vi "Mischer_LevelmeterMonitor.vi"() -> ()   [LabVIEW 2018]
uses:
  Utility/Monitor Communication/Mischer/Mischer_Levelmeter-Cluster.ctl
  Instrument_Setup.vi
  Global/Global Variables/Data_Display_global.vi
panel:
  in  "Stopp":bool
  in  "Mischer Levelmeter":T1={"Plot"=[], "N-Shield (%)"=0.0, "He (%)"=0.0, "Coldtrap (%)"=0.0, "He - POT (%)"=0.0, "N-Shield Refill"=FALSE, "Last fill Shield"="", "Auto Refill Shield"=TRUE, "Trap Refill"=FALSE, "Last fill Coldtrap"="", "Auto Refill Trap"=TRUE, "Shield Refill"=FALSE, "Coldtrap Refill"=FALSE, "Auto Trap activatet"=FALSE, "Auto Shield Activatet"=FALSE}
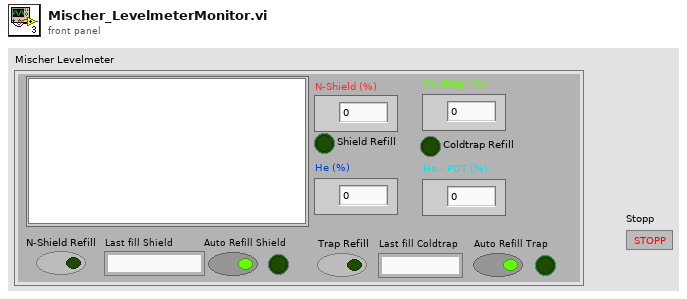
[diagram p1: front panel]
types:
  T1 = typedef "Mischer_Levelmeter-Cluster.ctl" = cluster{"Plot":dbl[][], "N-Shield (%)":dbl, "He (%)":dbl, "Coldtrap (%)":dbl, "He - POT (%)":dbl, "N-Shield Refill":bool, "Last fill Shield":string, "Auto Refill Shield":bool, "Trap Refill":bool, "Last fill Coldtrap":string, "Auto Refill Trap":bool, "Shield Refill":bool, "Coldtrap Refill":bool, "Auto Trap activatet":bool, "Auto Shield Activatet":bool}
  T2 = cluster{"Arduino Levelmeter":refnum<visa-resource-name>, "TIC Comport":refnum<visa-resource-name>}
  T3 = typedef "Mischer_Levelmeter_Control.ctl" = cluster{"N-Shield Refill":bool, "Automatic Refill Shield":bool, "Trap Refill":bool, "Automatic Refill Trap":bool}
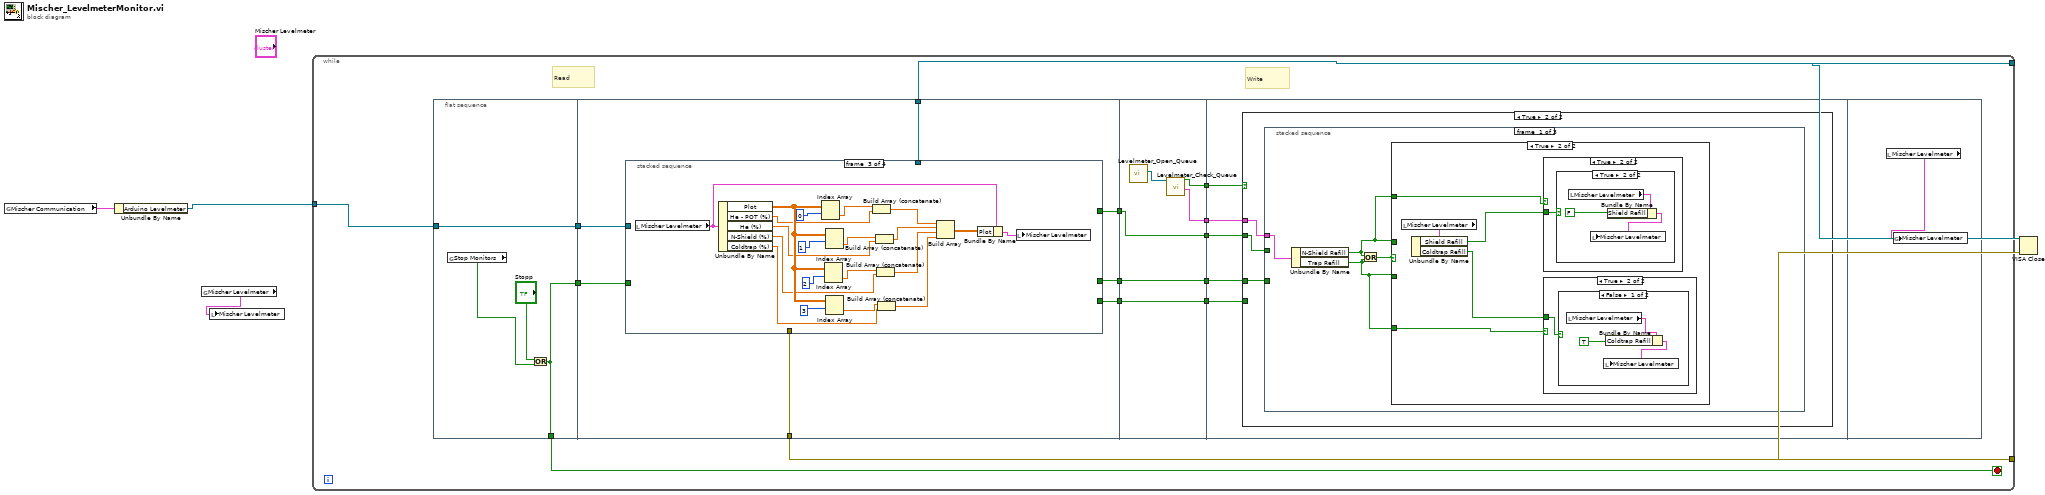
[diagram p0: block diagram]
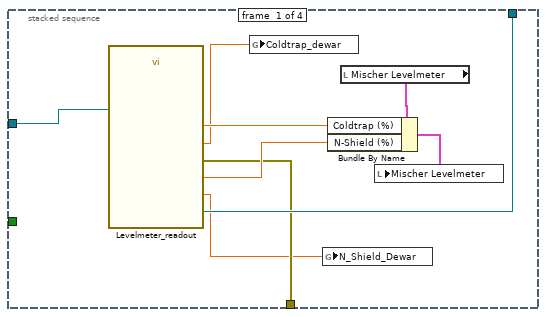
[diagram p2: hidden frame]
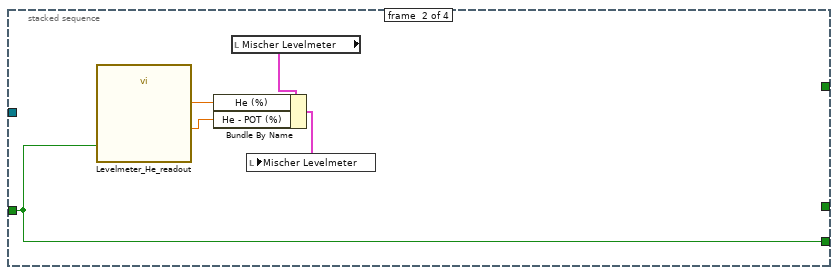
[diagram p3: hidden frame]
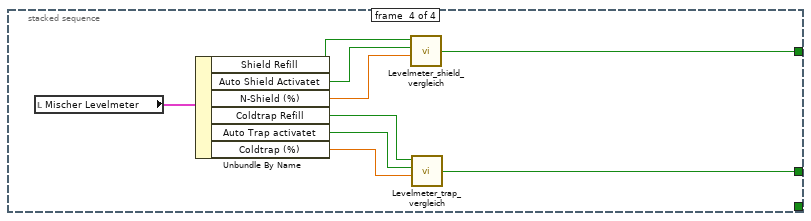
[diagram p4: hidden frame]
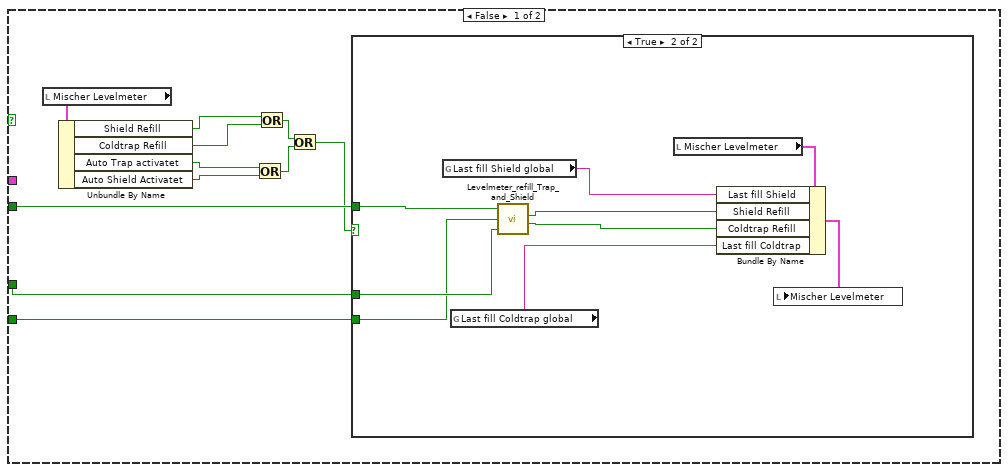
[diagram p5: hidden frame]
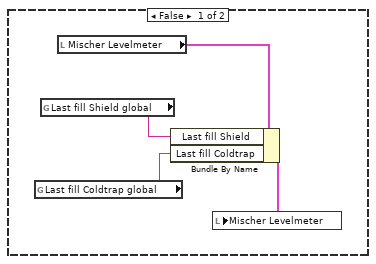
[diagram p6: hidden frame]
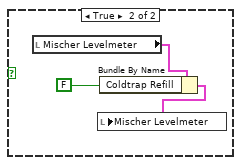
[diagram p9: hidden frame]
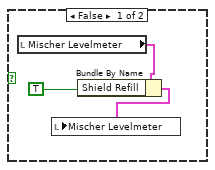
[diagram p11: hidden frame]
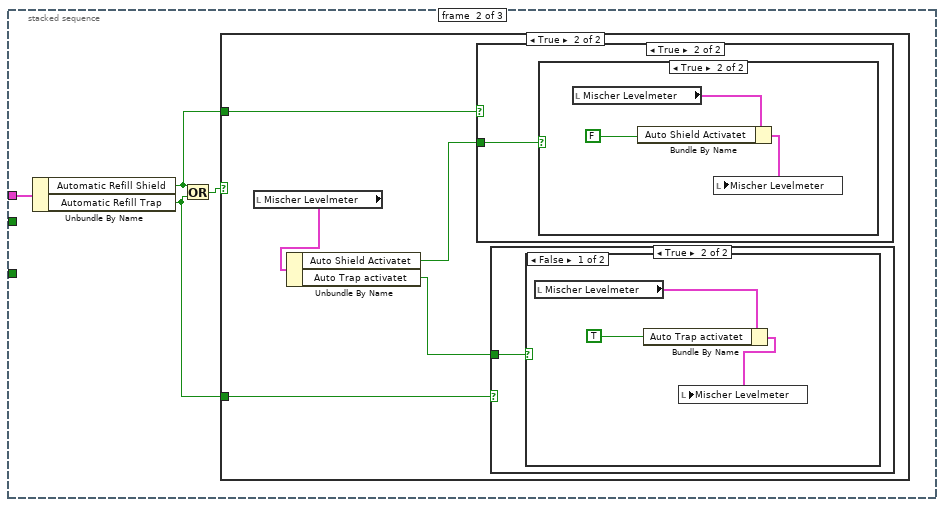
[diagram p12: hidden frame]
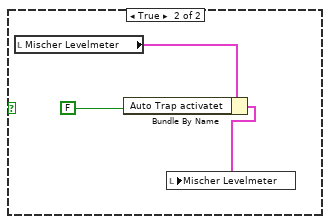
[diagram p15: hidden frame]
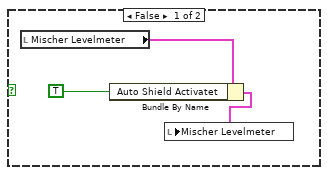
[diagram p17: hidden frame]
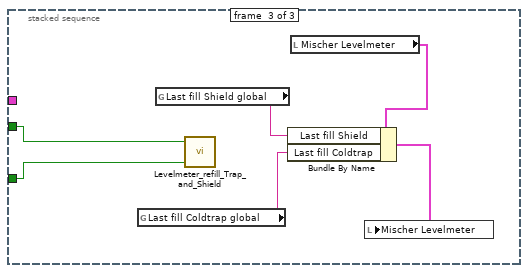
[diagram p18: hidden frame]
diagram:
  n1 = global read "Instrument_Setup.vi" "Mischer Communication"() -> (w5:T2)
  n2 = Unbundle By Name(w5) -> ("Arduino Levelmeter"=w1:refnum<visa-resource-name>)
  n3 = global read "Data_Display_global.vi" "Mischer Levelmeter"() -> (w4:T1)
  n4 = local write "Mischer Levelmeter"(w4) -> ()
  n5 = while {
    tunnel: w1 -> [w19]
    tunnel: [w12] -> w3
    tunnel: [w11] -> w2
    stop <- w9 stop-if-true
    # "Write"
    # "Read"
    n6 = flat-sequence {
      tunnel: w19 -> [w23]
      tunnel: [w23] -> w10
      tunnel: [w20] -> w9
      tunnel: [w20] -> w8
      tunnel: [w29] -> w16
      tunnel: [w28] -> w15
      tunnel: [w27] -> w12
      tunnel: [w26] -> w11
      tunnel: w10 -> [w30]
      tunnel: w8 -> [w25]
      tunnel: [w24] -> w6
      tunnel: [w78] -> w18
      tunnel: [w77] -> w17
      tunnel: w16 -> [w76]
      tunnel: w15 -> [w75]
      tunnel: [w76] -> w14
      tunnel: [w75] -> w13
      tunnel: [w74] -> w7
      tunnel: w6 -> [w74]
      tunnel: w18 -> [w83]
      tunnel: w17 -> [w84]
      tunnel: w14 -> [w82]
      tunnel: w13 -> [w81]
      tunnel: w7 -> [w80]
      frame #0 {
        n7 = global read "Data_Display_global.vi" "Stop Monitors"() -> (w22:bool)
        n8 = Or(x="Stopp", y=w22) -> (x .or. y?=w20:bool)
      }
      frame #1 {
        n9 = stacked-sequence {
          tunnel: w30 -> [w39 _ _ _]
          tunnel: [_ _ _ w65] -> w29
          tunnel: [_ _ _ w66] -> w28
          tunnel: [w34 _ _ _] -> w27
          tunnel: [w33 _ _ _] -> w26
          tunnel: w25 -> [_ w40 _ _]
          tunnel: [_ w40 _ _] -> w24
          frame #0 {
            n10 = call "Levelmeter_readout.vi"("VISA-Ressourcenname"=w39) -> ("LN Shield Dewar [%]"=w31:dbl, "Coldtrap Dewar [%]"=w32:dbl, "Cold trap [%]"=w36:dbl, "LN Shield [%]"=w35:dbl, "VISA-Ressourcenname 2"=w34:refnum<visa-resource-name>, "error out"=w33:errorcluster)  [unwired: 4 in]
            n11 = global write "Data_Display_global.vi" "Coldtrap_dewar"(w32) -> ()
            n12 = global write "Data_Display_global.vi" "N_Shield_Dewar"(w31) -> ()
            n13 = local read "Mischer Levelmeter"() -> (w38:T1)
            n14 = Bundle By Name(cluster=w38, "Coldtrap (%)"=w36, "N-Shield (%)"=w35) -> (w37:T1)
            n15 = local write "Mischer Levelmeter"(w37) -> ()
          }
          frame #1 {
            n16 = call "Levelmeter_He_readout.vi"("stop DAQ"=w40) -> ("He-Pot in (%)"=w41:dbl, "He Bath (%)"=w44:dbl)  [unwired: 9 in]
            n17 = local read "Mischer Levelmeter"() -> (w43:T1)
            n18 = Bundle By Name(cluster=w43, "He (%)"=w44, "He - POT (%)"=w41) -> (w42:T1)
            n19 = local write "Mischer Levelmeter"(w42) -> ()
          }
          frame #2 {
            n20 = local read "Mischer Levelmeter"() -> (w47:T1)
            n21 = Unbundle By Name(w47) -> ("Plot"=w64:dbl[][], "He - POT (%)"=w58:dbl, "He (%)"=w56:dbl, "N-Shield (%)"=w54:dbl, "Coldtrap (%)"=w52:dbl)
            n22 = Index Array(array=w64, index (row)=0) -> (element=w59:dbl[])  [unwired: 1 in]
            n23 = Index Array(array=w64, index (row)=2) -> (element=w55:dbl[])  [unwired: 1 in]
            n24 = Index Array(array=w64, index (row)=1) -> (element=w57:dbl[])  [unwired: 1 in]
            n25 = Index Array(array=w64, index (row)=3) -> (element=w53:dbl[])  [unwired: 1 in]
            n26 = Build Array (concatenate)(w59, w58) -> (w51:dbl[])
            n27 = Build Array (concatenate)(w57, w56) -> (w50:dbl[])
            n28 = Build Array (concatenate)(w55, w54) -> (w49:dbl[])
            n29 = Build Array (concatenate)(w53, w52) -> (w48:dbl[])
            n30 = Build Array(w51, w50, w49, w48) -> (w46:dbl[][])
            n31 = Bundle By Name(cluster=w47, "Plot"=w46) -> (w45:T1)
            n32 = local write "Mischer Levelmeter"(w45) -> ()
          }
          frame #3 {
            n33 = local read "Mischer Levelmeter"() -> (w67:T1)
            n34 = Unbundle By Name(w67) -> ("Shield Refill"=w73:bool, "Auto Shield Activatet"=w72:bool, "N-Shield (%)"=w71:dbl, "Coldtrap Refill"=w70:bool, "Auto Trap activatet"=w69:bool, "Coldtrap (%)"=w68:dbl)
            n35 = call "Levelmeter_shield_vergleich.vi"("Shield Level (%)"=w71, "Automatic Shield refill activatet"=w72, "LN Shield Refill activatet"=w73) -> ("Data out"=w65:bool)  [unwired: 3 in]
            n36 = call "Levelmeter_trap_vergleich.vi"("Coldtrap Level (%)"=w68, "Automatic Trap refill activatet"=w69, "LN trap Refill activatet"=w70) -> ("Data out"=w66:bool)  [unwired: 3 in]
          }
        }
      }
      frame #2 {
        n37 = call "Levelmeter_Open_Queue.vi"() -> ("queue out"=w79:refnum<queue>)  [unwired: 10 in, 1 out]
        n38 = call "Levelmeter_Check_Queue.vi"("queue"=w79) -> ("Mischer Levelmeter  Control"=w78:T3, "New Entries?"=w77:bool)  [unwired: 7 in, 1 out]
      }
      frame #3 {
        n39 = case shown="True" w84 {
          tunnel: w83 -> [_ w111]
          tunnel: w82 -> [w95 w110]
          tunnel: w81 -> [w94 w109]
          tunnel: w80 -> [w85 _]
          frame False {
            n40 = local read "Mischer Levelmeter"() -> (w93:T1)
            n41 = Unbundle By Name(w93) -> ("Shield Refill"=w92:bool, "Coldtrap Refill"=w91:bool, "Auto Trap activatet"=w90:bool, "Auto Shield Activatet"=w89:bool)
            n42 = Or(x=w90, y=w89) -> (x .or. y?=w87:bool)
            n43 = Or(x=w92, y=w91) -> (x .or. y?=w88:bool)
            n44 = Or(x=w88, y=w87) -> (x .or. y?=w86:bool)
            n45 = case shown="True" w86 {
              tunnel: w95 -> [_ w108]
              tunnel: w94 -> [_ w107]
              tunnel: w85 -> [_ w100]
              frame False {
                n46 = global read "Data_Display_global.vi" "Last fill Coldtrap global"() -> (w96:string)
                n47 = global read "Data_Display_global.vi" "Last fill Shield global"() -> (w97:string)
                n48 = local read "Mischer Levelmeter"() -> (w99:T1)
                n49 = Bundle By Name(cluster=w99, "Last fill Shield"=w97, "Last fill Coldtrap"=w96) -> (w98:T1)
                n50 = local write "Mischer Levelmeter"(w98) -> ()
              }
              frame True {
                n51 = global read "Data_Display_global.vi" "Last fill Shield global"() -> (w102:string)
                n52 = global read "Data_Display_global.vi" "Last fill Coldtrap global"() -> (w101:string)
                n53 = call "Levelmeter_refill_Trap_and_Shield.vi"("Shield Refill"=w108, "Stop DAQ"=w100, "Trap Refill"=w107) -> ("Shield control"=w105:bool, "Trap control"=w104:bool)  [unwired: 2 in]
                n54 = local read "Mischer Levelmeter"() -> (w106:T1)
                n55 = Bundle By Name(cluster=w106, "Last fill Shield"=w102, "Shield Refill"=w105, "Coldtrap Refill"=w104, "Last fill Coldtrap"=w101) -> (w103:T1)
                n56 = local write "Mischer Levelmeter"(w103) -> ()
              }
            }
          }
          frame True {
            n57 = stacked-sequence {
              tunnel: w111 -> [w114 w138 _]
              tunnel: w110 -> [_ _ w163]
              tunnel: w109 -> [_ _ w162]
              frame #0 {
                n58 = Unbundle By Name(w114) -> ("N-Shield Refill"=w113:bool, "Trap Refill"=w112:bool)
                n59 = Or(x=w113, y=w112) -> (x .or. y?=w115:bool)
                n60 = case shown="True" w115 {
                  tunnel: w113 -> [_ _]
                  tunnel: w112 -> [_ _]
                  tunnel: w113 -> [_ w119]
                  tunnel: w112 -> [_ w118]
                  frame False {
                  }
                  frame True {
                    n61 = local read "Mischer Levelmeter"() -> (w120:T1)
                    n62 = Unbundle By Name(w120) -> ("Shield Refill"=w117:bool, "Coldtrap Refill"=w116:bool)
                    n63 = case shown="True" w119 {
                      tunnel: w117 -> [_ w128]
                      frame False {
                      }
                      frame True {
                        n64 = case shown="True" w128 {
                          frame False {
                            n65 = local read "Mischer Levelmeter"() -> (w131:T1)
                            n66 = Bundle By Name(cluster=w131, "Shield Refill"=TRUE) -> (w130:T1)
                            n67 = local write "Mischer Levelmeter"(w130) -> ()
                          }
                          frame True {
                            n68 = local read "Mischer Levelmeter"() -> (w134:T1)
                            n69 = Bundle By Name(cluster=w134, "Shield Refill"=FALSE) -> (w133:T1)
                            n70 = local write "Mischer Levelmeter"(w133) -> ()
                          }
                        }
                      }
                    }
                    n71 = case shown="True" w118 {
                      tunnel: w116 -> [_ w121]
                      frame False {
                      }
                      frame True {
                        n72 = case shown="False" w121 {
                          frame False {
                            n73 = local read "Mischer Levelmeter"() -> (w124:T1)
                            n74 = Bundle By Name(cluster=w124, "Coldtrap Refill"=TRUE) -> (w123:T1)
                            n75 = local write "Mischer Levelmeter"(w123) -> ()
                          }
                          frame True {
                            n76 = local read "Mischer Levelmeter"() -> (w127:T1)
                            n77 = Bundle By Name(cluster=w127, "Coldtrap Refill"=FALSE) -> (w126:T1)
                            n78 = local write "Mischer Levelmeter"(w126) -> ()
                          }
                        }
                      }
                    }
                  }
                }
              }
              frame #1 {
                n79 = Unbundle By Name(w138) -> ("Automatic Refill Shield"=w136:bool, "Automatic Refill Trap"=w135:bool)
                n80 = Or(x=w136, y=w135) -> (x .or. y?=w137:bool)
                n81 = case shown="True" w137 {
                  tunnel: w136 -> [_ w140]
                  tunnel: w135 -> [_ w139]
                  frame False {
                  }
                  frame True {
                    n82 = local read "Mischer Levelmeter"() -> (w143:T1)
                    n83 = Unbundle By Name(w143) -> ("Auto Shield Activatet"=w142:bool, "Auto Trap activatet"=w141:bool)
                    n84 = case shown="True" w140 {
                      tunnel: w142 -> [_ w151]
                      frame False {
                      }
                      frame True {
                        n85 = case shown="True" w151 {
                          frame False {
                            n86 = local read "Mischer Levelmeter"() -> (w154:T1)
                            n87 = Bundle By Name(cluster=w154, "Auto Shield Activatet"=TRUE) -> (w152:T1)
                            n88 = local write "Mischer Levelmeter"(w152) -> ()
                          }
                          frame True {
                            n89 = local read "Mischer Levelmeter"() -> (w157:T1)
                            n90 = Bundle By Name(cluster=w157, "Auto Shield Activatet"=FALSE) -> (w155:T1)
                            n91 = local write "Mischer Levelmeter"(w155) -> ()
                          }
                        }
                      }
                    }
                    n92 = case shown="True" w139 {
                      tunnel: w141 -> [_ w144]
                      frame False {
                      }
                      frame True {
                        n93 = case shown="False" w144 {
                          frame False {
                            n94 = local read "Mischer Levelmeter"() -> (w147:T1)
                            n95 = Bundle By Name(cluster=w147, "Auto Trap activatet"=TRUE) -> (w145:T1)
                            n96 = local write "Mischer Levelmeter"(w145) -> ()
                          }
                          frame True {
                            n97 = local read "Mischer Levelmeter"() -> (w150:T1)
                            n98 = Bundle By Name(cluster=w150, "Auto Trap activatet"=FALSE) -> (w148:T1)
                            n99 = local write "Mischer Levelmeter"(w148) -> ()
                          }
                        }
                      }
                    }
                  }
                }
              }
              frame #2 {
                n100 = global read "Data_Display_global.vi" "Last fill Coldtrap global"() -> (w160:string)
                n101 = global read "Data_Display_global.vi" "Last fill Shield global"() -> (w161:string)
                n102 = call "Levelmeter_refill_Trap_and_Shield.vi"("Shield Refill"=w163, "Trap Refill"=w162) -> ()  [unwired: 3 in, 2 out]
                n103 = local read "Mischer Levelmeter"() -> (w159:T1)
                n104 = Bundle By Name(cluster=w159, "Last fill Shield"=w161, "Last fill Coldtrap"=w160) -> (w158:T1)
                n105 = local write "Mischer Levelmeter"(w158) -> ()
              }
            }
          }
        }
      }
      frame #4 {
        n106 = local read "Mischer Levelmeter"() -> (w164:T1)
        n107 = global write "Data_Display_global.vi" "Mischer Levelmeter"(w164) -> ()
      }
    }
  }
  n108 = VISA Close(VISA resource name=w3, error in (no error)=w2) -> ()  [unwired: 1 out]
